vi "Finish Create.vi"(4 "Actor Ref":refnum<vi>, 5 "Alias":string, 6 "Creator Attributes":refnum<class "Attributes.lvclass">, 7 "Unified Msg Set":T1, 10 "Queue of Self Attributes":refnum<queue>, 11 "Base Actor in":refnum<class "Base Actor.lvclass">) -> (0 "Error out":errorcluster, 3 "Base Actor out":refnum<class "Base Actor.lvclass">)   [LabVIEW 2020, in "jettl.lvlib" / "Actor.lvlib" / "Base Actor.lvclass"]
uses:
  Base Actor.lvclass
  Attributes/Attributes/Attributes.lvclass
  Msg Set.ctl
  Msg/Msg.lvclass
  Base Actor.lvclass/Base Actor.ctl
  Attributes/Attributes.lvlib
  Actor.lvlib
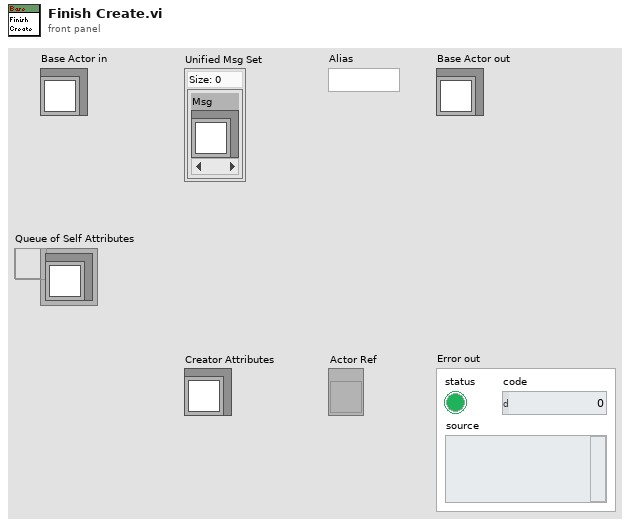
[diagram p1: front panel]
types:
  T1 = typedef "jettl.lvlib/Actor.lvlib/Msg Set.ctl" = set{refnum<class "Msg.lvclass">}
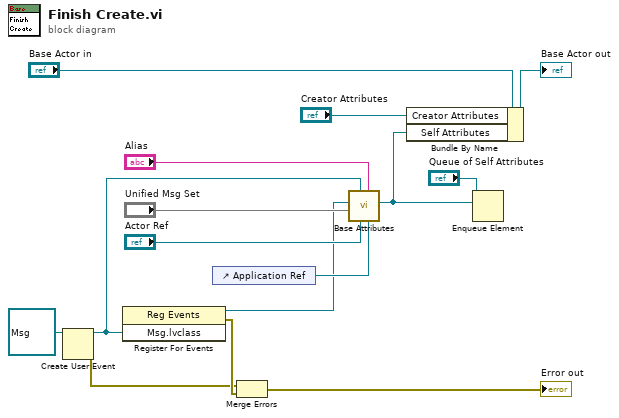
[diagram p0: block diagram]
diagram:
  n1 = Create User Event(user event datatype=refnum<class "Msg.lvclass"> refnum ("Msg.lvclass")) -> (user event=w6:refnum<user-event>, error out=w13:errorcluster)  [unwired: 1 in]
  n2 = register-events(w6) -> (reference out=w5:refnum<event-registration>, error out=w14:errorcluster)  [unwired: 2 in]
  n3 = control-ref of="Application Ref"() -> (w10:refnum<vi>)
  n4 = Merge Errors(w13, w14) -> (→"Error out":errorcluster)
  n5 = call "Base Attributes.vi"("Application Ref"=w10, "Alias"="Alias", "Actor Ref"="Actor Ref", "Address"=w6, "Unified Msg Set"="Unified Msg Set", "Event Ref"=w5) -> ("Attributes"=w2:refnum<class "Attributes.lvclass">)  [unwired: 5 in]
  n6 = Bundle By Name(cluster="Base Actor in", "Creator Attributes"="Creator Attributes", "Self Attributes"=w2) -> (→"Base Actor out":refnum<class "Base Actor.lvclass">)
  n7 = Enqueue Element(queue="Queue of Self Attributes", element=w2) -> ()  [unwired: 2 in, 3 out]
